vi "CRC16 CCITT False.vi"(8 "error in (no error)":errorcluster, 11 "data":u8[](array[numeric])) -> (0 "error out":errorcluster, 3 "crc":u8[](array[numeric]))   [LabVIEW 2023]
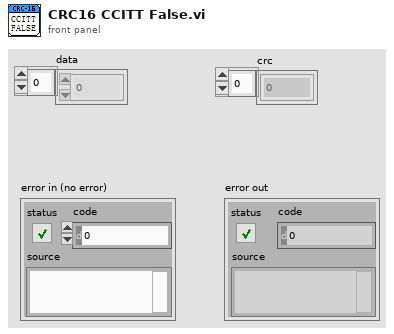
[diagram p1: front panel]
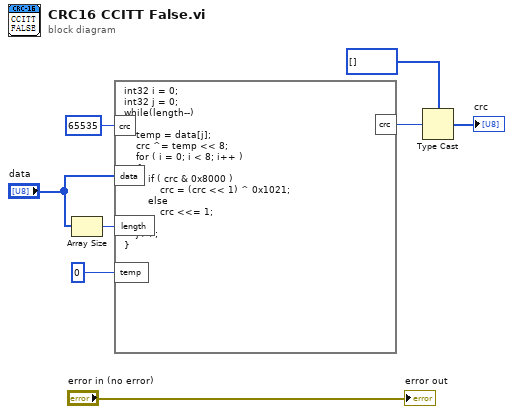
[diagram p0: block diagram]
diagram:
  n1 = Array Size(array="data") -> (size(s)=w8:i32)
  n2 = formula code="int32 i = 0;\nint32 j = 0;\nwhile(length--)\n{\n    temp = data[j];\n    crc ^= temp << 8; \n    for ( i = 0; i < 8; i++ )\n    {\n        if ( crc & 0x8000 )\n            crc = (crc << 1) ^ 0x1021;\n        else\n            crc <<= 1;\n    }\n    j++;\n}"("data"="data", "length"=w8, "crc"=u16 65535, "temp"=u16 0) -> ("crc"=w6:u16)
  n3 = Type Cast(type=u8[] [] ("unsigned byte array"), x=w6) -> (*(type *) &x=→"crc":u8[])
  "error out" <- "error in (no error)"
